vi "PicoScope5000aSettings.vi"(0 "error in":errorcluster, 1 "Channel A Settings":T2={"Enabled"=FALSE, "Coupling"=1, "Range"=6, "Analogue Offset"=0.0, "Bandwidth Limit"=0} {"Bandwidth Limit" items=["Full", "20MHz"]; "Range" items=["10 mV", "20 mV", "50 mV", "100 mV", "200 mV", "500 mV", "1 V", "2 V", "5 V", "10 V", "20 V"]; "Coupling" items=["AC", "DC"]}, 2 "Port 0 Settings":cluster{"Enabled":bool, "Logic Level":i16}={"Enabled"=FALSE, "Logic Level"=9830} {"Logic Level" items=["1.5V TTL"=9830, "2.5V CMOS"=16383]}, 3 "Channel B Settings":T2={"Enabled"=FALSE, "Coupling"=1, "Range"=6, "Analogue Offset"=0.0, "Bandwidth Limit"=0} {"Bandwidth Limit" items=["Full", "20MHz"]; "Range" items=["10 mV", "20 mV", "50 mV", "100 mV", "200 mV", "500 mV", "1 V", "2 V", "5 V", "10 V", "20 V"]; "Coupling" items=["AC", "DC"]}, 5 "handle in":i16, 9 "Device Info":T1, 11 "Trigger Settings":T3={"Trigger Enabled"=FALSE, "Trigger Source"=enum."Channel A", "Trigger Threshold (volts)"=0.0, "Trigger Direction"=2, "Trigger Delay (samples)"=0, "Auto Trigger Time (ms)"=1000} {"Trigger Direction" items=["Rising"=2, "Falling"=3]}, 12 "Channel C Settings":T2={"Enabled"=FALSE, "Coupling"=1, "Range"=6, "Analogue Offset"=0.0, "Bandwidth Limit"=0} {"Bandwidth Limit" items=["Full", "20MHz"]; "Range" items=["10 mV", "20 mV", "50 mV", "100 mV", "200 mV", "500 mV", "1 V", "2 V", "5 V", "10 V", "20 V"]; "Coupling" items=["AC", "DC"]}, 13 "Port 1 Settings":cluster{"Enabled":bool, "Logic Level":i16}={"Enabled"=FALSE, "Logic Level"=9830} {"Logic Level" items=["1.5V TTL"=9830, "2.5V CMOS"=16383]}, 14 "Channel D Settings":T2={"Enabled"=FALSE, "Coupling"=1, "Range"=6, "Analogue Offset"=0.0, "Bandwidth Limit"=0} {"Bandwidth Limit" items=["Full", "20MHz"]; "Range" items=["10 mV", "20 mV", "50 mV", "100 mV", "200 mV", "500 mV", "1 V", "2 V", "5 V", "10 V", "20 V"]; "Coupling" items=["AC", "DC"]}, 15 "Max ADC value":i16) -> (4 "error out":errorcluster, 6 "handle out":i16, 8 "enabled array":i16[](array[numeric]))   [LabVIEW 2020]
doc: "This VI is used to set up the oscilloscope. The inputs are clusters for setting channel and simple trigger settings. Advanced triggers can be set up using PicoScope3000aAdvancedTriggerSettings.vi"
uses:
  ps5000a.dll
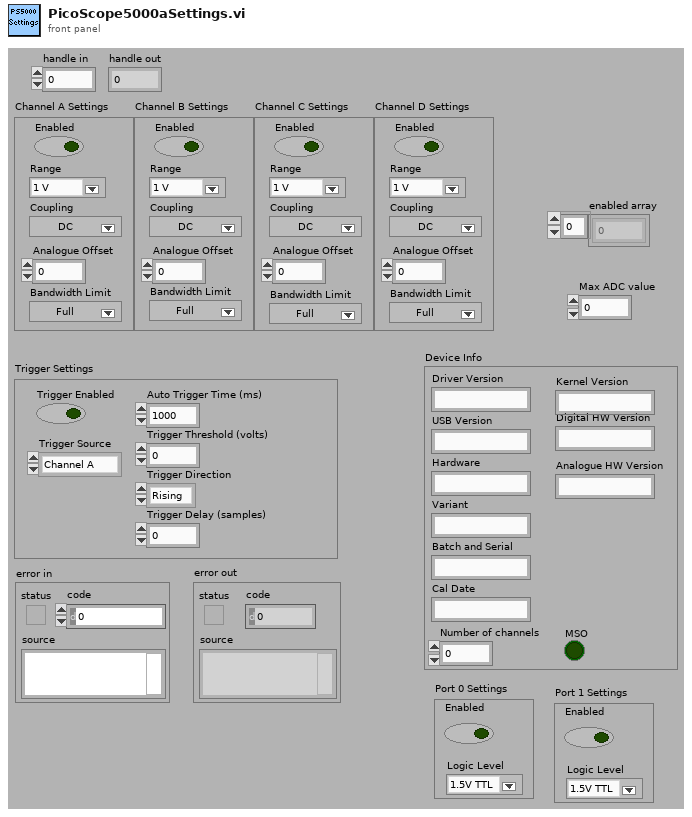
[diagram p1: front panel]
types:
  T1 = cluster{"Driver Version":string, "USB Version":string, "Hardware":string, "Variant":string, "Batch and Serial":string, "Cal Date":string, "Kernel Version":string, "Digital HW Version":string, "Analogue HW Version":string, "MSO":bool, "Number of channels":i16}
  T2 = cluster{"Enabled":bool, "Coupling":i16, "Range":u16, "Analogue Offset":sgl, "Bandwidth Limit":u32}
  T3 = cluster{"Trigger Enabled":bool, "Trigger Source":enum16{"Channel A", "Channel B", "Channel C", "Channel D", "Ext."}, "Trigger Threshold (volts)":dbl, "Trigger Direction":u16, "Trigger Delay (samples)":u32, "Auto Trigger Time (ms)":i16}
  T4 = enum16{"Channel A", "Channel B", "Channel C", "Channel D", "Ext."}
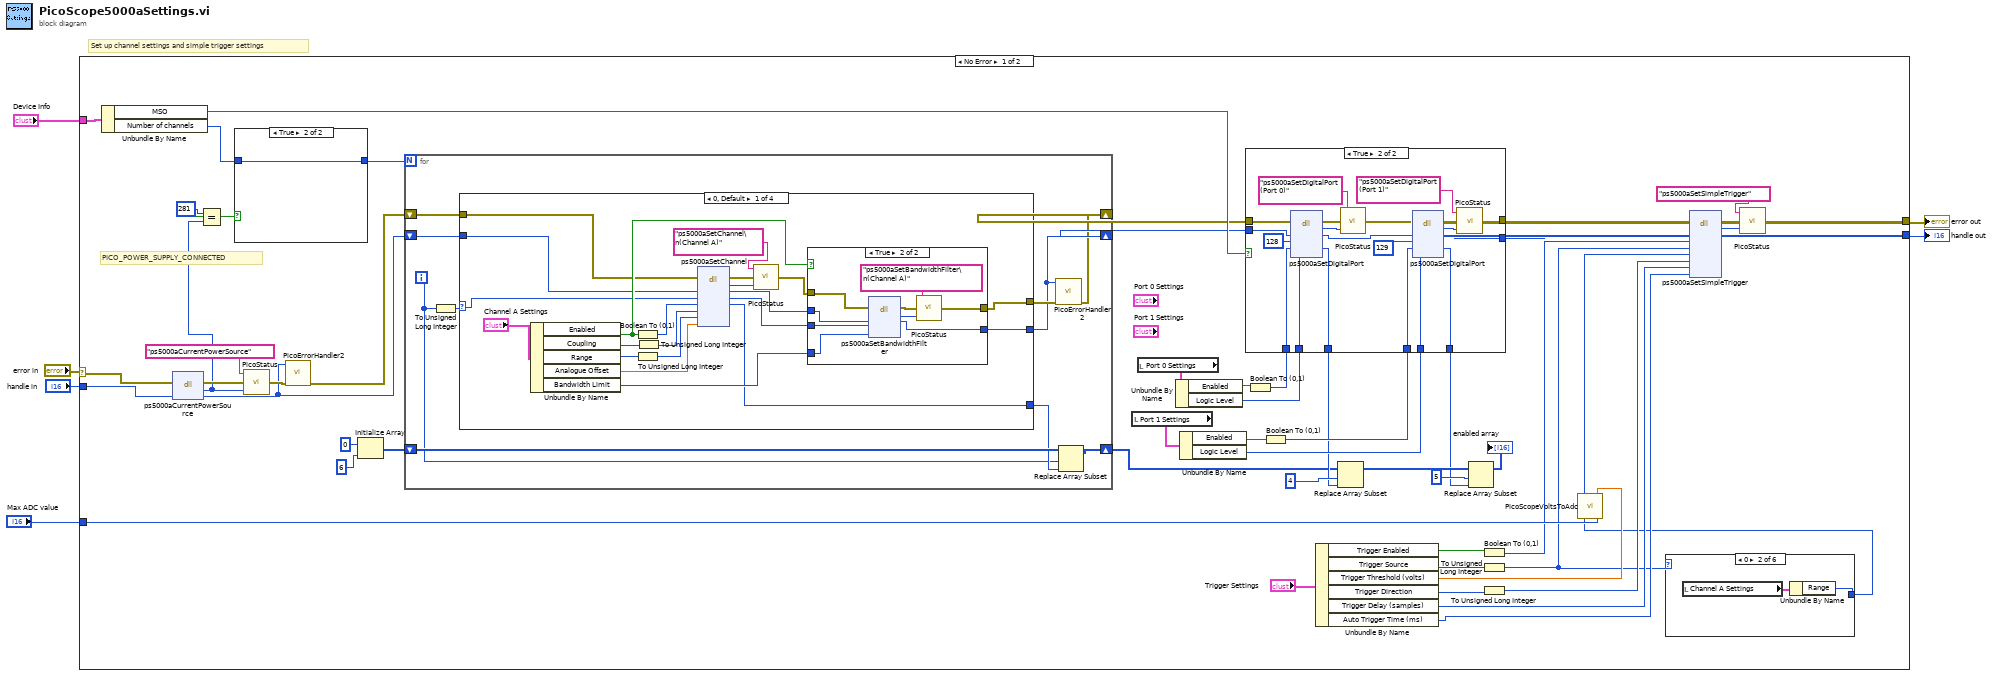
[diagram p0: block diagram]
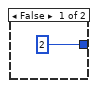
[diagram p2: hidden frame]
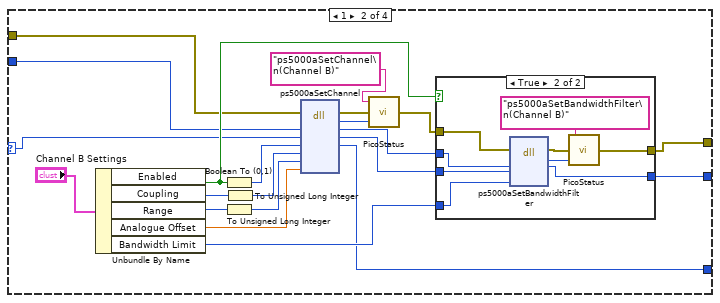
[diagram p4: hidden frame]
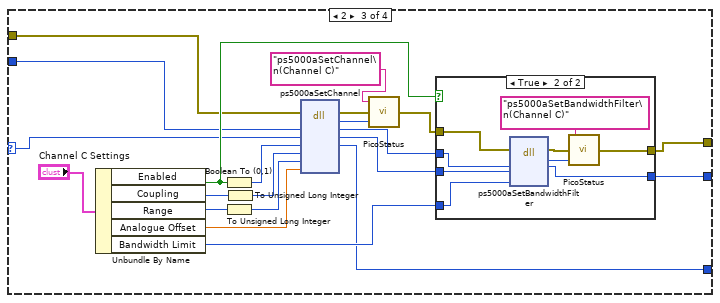
[diagram p6: hidden frame]
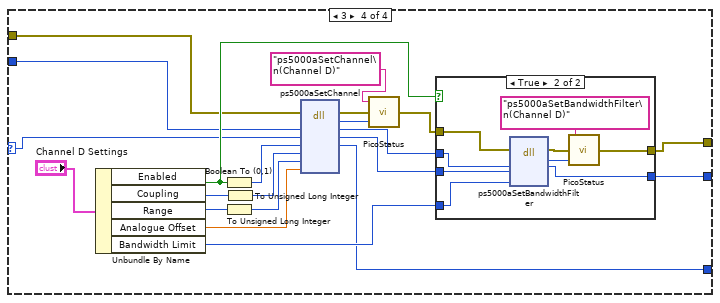
[diagram p8: hidden frame]
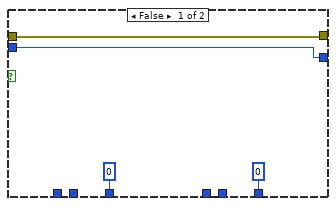
[diagram p10: hidden frame]
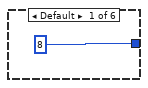
[diagram p11: hidden frame]
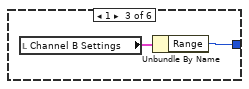
[diagram p12: hidden frame]
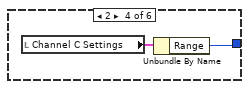
[diagram p13: hidden frame]
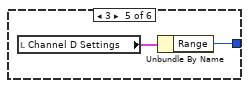
[diagram p14: hidden frame]
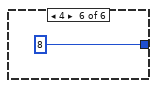
[diagram p15: hidden frame]
diagram:
  # "Set up channel settings and simple trigger settings"
  n1 = case shown="No Error" "error in" {
    selector: "error in" -> [w15 w236]
    tunnel: "handle in" -> [w14 w235]
    tunnel: [w51 w235] -> w4
    tunnel: [w40 w236] -> w3
    tunnel: "Device Info" -> [w46 _]
    tunnel: "Max ADC value" -> [w43 _]
    frame No Error {
      # "PICO_POWER_SUPPLY_CONNECTED"
      n2 = Unbundle By Name(w46) -> ("MSO"=w22:bool, "Number of channels"=w8:i16)
      n3 = dll-call lib="ps5000a.dll" fn="ps5000aCurrentPowerSource"(error in=w15, "handle"=w14) -> (error out=w49:errorcluster, "PICO_STATUS"=w47:u32, "handle"=w12:i16)  [unwired: 2 in, 1 out]
      n4 = Equal?(x=u32 281, y=w47) -> (x = y?=w10:bool)
      n5 = case shown="True" w10 {
        tunnel: [i16 2 ("Number of channels") w62] -> w9
        tunnel: w8 -> [_ w62]
        frame False {
        }
        frame True {
        }
      }
      n6 = call "PicoStatus.vi"("PICO STATUS"=w47, "error in"=w49, "source"="ps5000aCurrentPowerSource") -> ("error out"=w13:errorcluster)
      n7 = call "PicoErrorHandler2.vi"("error in (no error)"=w13, "handle In"=w12) -> ("error out"=w11:errorcluster)  [unwired: 9 in]
      n8 = Initialize Array(i16 0 ("element"), 6 ("dimension size")) -> (w19:i16[])
      n9 = for {
        N: w9 -> [_]
        shift-right: [w70] -> w18
        shift-left: w19 -> [w72]
        shift-right: [w67] -> w17
        shift-left: w11 -> [w69]
        shift-right: [w65] -> w16
        shift-left: w12 -> [w68]
        i -> [w63]
        n10 = To Unsigned Long Integer(number=w63) -> (unsigned 32bit integer=w64:u32)
        n11 = case shown="0, Default" w64 {
          selector: w64 -> [w73 w105 w137 w169]
          tunnel: [w78 w111 w143 w175] -> w71
          tunnel: w69 -> [w77 w109 w141 w173]
          tunnel: w68 -> [w76 w108 w140 w172]
          tunnel: [w75 w107 w139 w171] -> w66
          tunnel: [w74 w106 w138 w170] -> w65
          frame 0, Default {
            n12 = Unbundle By Name("Channel A Settings") -> ("Enabled"=w82:bool, "Coupling"=w92:i16, "Range"=w93:u16, "Analogue Offset"=w90:sgl, "Bandwidth Limit"=w83:u32)
            n13 = Boolean To (0,1)(Boolean=w82) -> (0, 1=w85:i16)
            n14 = To Unsigned Long Integer(number=w93) -> (unsigned 32bit integer=w89:u32)
            n15 = To Unsigned Long Integer(number=w92) -> (unsigned 32bit integer=w91:u32)
            n16 = dll-call lib="ps5000a.dll" fn="ps5000aSetChannel" ("ps3000.dll:_ps3000_open_unit@0")(error in=w77, "handle"=w76, "channel"=w73, "enabled"=w85, "dc"=w91, "range"=w89, "analogueOffset"=w90) -> (error out=w88:errorcluster, "PICO_STATUS"=w87:u32, "handle"=w80:i16, "channel"=w79:u32, "enabled"=w78:i16)  [unwired: 5 in, 1 out]
            n17 = call "PicoStatus.vi"("PICO STATUS"=w87, "error in"=w88, "source"="ps5000aSetChannel\n(Channel A)") -> ("error out"=w81:errorcluster)
            n18 = case shown="True" w82 {
              tunnel: w81 -> [w95 w101]
              tunnel: [w95 w100] -> w75
              tunnel: [w94 w99] -> w74
              tunnel: w79 -> [_ w98]
              tunnel: w80 -> [w94 w97]
              tunnel: w83 -> [_ w96]
              frame False {
              }
              frame True {
                n19 = dll-call lib="ps5000a.dll" fn="ps5000aSetBandwidthFilter" ("ps3000.dll:_ps3000_open_unit@0")(error in=w101, "handle"=w97, "channel"=w98, "Bandwidth Limit"=w96) -> (error out=w103:errorcluster, "PICO_STATUS"=w102:u32, "handle"=w99:i16)  [unwired: 4 in, 1 out]
                n20 = call "PicoStatus.vi"("PICO STATUS"=w102, "error in"=w103, "source"="ps5000aSetBandwidthFilter\n(Channel A)") -> ("error out"=w100:errorcluster)
              }
            }
          }
          frame 1 {
            n21 = Unbundle By Name("Channel B Settings") -> ("Enabled"=w115:bool, "Coupling"=w124:i16, "Range"=w125:u16, "Analogue Offset"=w122:sgl, "Bandwidth Limit"=w116:u32)
            n22 = Boolean To (0,1)(Boolean=w115) -> (0, 1=w118:i16)
            n23 = To Unsigned Long Integer(number=w125) -> (unsigned 32bit integer=w121:u32)
            n24 = To Unsigned Long Integer(number=w124) -> (unsigned 32bit integer=w123:u32)
            n25 = dll-call lib="ps5000a.dll" fn="ps5000aSetChannel" ("ps3000.dll:_ps3000_open_unit@0")(error in=w109, "handle"=w108, "channel"=w105, "enabled"=w118, "dc"=w123, "range"=w121, "analogueOffset"=w122) -> (error out=w120:errorcluster, "PICO_STATUS"=w119:u32, "handle"=w113:i16, "channel"=w112:u32, "enabled"=w111:i16)  [unwired: 5 in, 1 out]
            n26 = call "PicoStatus.vi"("PICO STATUS"=w119, "error in"=w120, "source"="ps5000aSetChannel\n(Channel B)") -> ("error out"=w114:errorcluster)
            n27 = case shown="True" w115 {
              tunnel: w114 -> [w127 w133]
              tunnel: [w127 w132] -> w107
              tunnel: [w126 w131] -> w106
              tunnel: w112 -> [_ w130]
              tunnel: w113 -> [w126 w129]
              tunnel: w116 -> [_ w128]
              frame False {
              }
              frame True {
                n28 = dll-call lib="ps5000a.dll" fn="ps5000aSetBandwidthFilter" ("ps3000.dll:_ps3000_open_unit@0")(error in=w133, "handle"=w129, "channel"=w130, "Bandwidth Limit"=w128) -> (error out=w135:errorcluster, "PICO_STATUS"=w134:u32, "handle"=w131:i16)  [unwired: 4 in, 1 out]
                n29 = call "PicoStatus.vi"("PICO STATUS"=w134, "error in"=w135, "source"="ps5000aSetBandwidthFilter\n(Channel B)") -> ("error out"=w132:errorcluster)
              }
            }
          }
          frame 2 {
            n30 = Unbundle By Name("Channel C Settings") -> ("Enabled"=w147:bool, "Coupling"=w156:i16, "Range"=w157:u16, "Analogue Offset"=w154:sgl, "Bandwidth Limit"=w148:u32)
            n31 = Boolean To (0,1)(Boolean=w147) -> (0, 1=w150:i16)
            n32 = To Unsigned Long Integer(number=w157) -> (unsigned 32bit integer=w153:u32)
            n33 = To Unsigned Long Integer(number=w156) -> (unsigned 32bit integer=w155:u32)
            n34 = dll-call lib="ps5000a.dll" fn="ps5000aSetChannel" ("ps3000.dll:_ps3000_open_unit@0")(error in=w141, "handle"=w140, "channel"=w137, "enabled"=w150, "dc"=w155, "range"=w153, "analogueOffset"=w154) -> (error out=w152:errorcluster, "PICO_STATUS"=w151:u32, "handle"=w145:i16, "channel"=w144:u32, "enabled"=w143:i16)  [unwired: 5 in, 1 out]
            n35 = call "PicoStatus.vi"("PICO STATUS"=w151, "error in"=w152, "source"="ps5000aSetChannel\n(Channel C)") -> ("error out"=w146:errorcluster)
            n36 = case shown="True" w147 {
              tunnel: w146 -> [w159 w165]
              tunnel: [w159 w164] -> w139
              tunnel: [w158 w163] -> w138
              tunnel: w144 -> [_ w162]
              tunnel: w145 -> [w158 w161]
              tunnel: w148 -> [_ w160]
              frame False {
              }
              frame True {
                n37 = dll-call lib="ps5000a.dll" fn="ps5000aSetBandwidthFilter" ("ps3000.dll:_ps3000_open_unit@0")(error in=w165, "handle"=w161, "channel"=w162, "Bandwidth Limit"=w160) -> (error out=w167:errorcluster, "PICO_STATUS"=w166:u32, "handle"=w163:i16)  [unwired: 4 in, 1 out]
                n38 = call "PicoStatus.vi"("PICO STATUS"=w166, "error in"=w167, "source"="ps5000aSetBandwidthFilter\n(Channel C)") -> ("error out"=w164:errorcluster)
              }
            }
          }
          frame 3 {
            n39 = Unbundle By Name("Channel D Settings") -> ("Enabled"=w179:bool, "Coupling"=w188:i16, "Range"=w189:u16, "Analogue Offset"=w186:sgl, "Bandwidth Limit"=w180:u32)
            n40 = Boolean To (0,1)(Boolean=w179) -> (0, 1=w182:i16)
            n41 = To Unsigned Long Integer(number=w189) -> (unsigned 32bit integer=w185:u32)
            n42 = To Unsigned Long Integer(number=w188) -> (unsigned 32bit integer=w187:u32)
            n43 = dll-call lib="ps5000a.dll" fn="ps5000aSetChannel" ("ps3000.dll:_ps3000_open_unit@0")(error in=w173, "handle"=w172, "channel"=w169, "enabled"=w182, "dc"=w187, "range"=w185, "analogueOffset"=w186) -> (error out=w184:errorcluster, "PICO_STATUS"=w183:u32, "handle"=w177:i16, "channel"=w176:u32, "enabled"=w175:i16)  [unwired: 5 in, 1 out]
            n44 = call "PicoStatus.vi"("PICO STATUS"=w183, "error in"=w184, "source"="ps5000aSetChannel\n(Channel D)") -> ("error out"=w178:errorcluster)
            n45 = case shown="True" w179 {
              tunnel: w178 -> [w191 w197]
              tunnel: [w191 w196] -> w171
              tunnel: [w190 w195] -> w170
              tunnel: w176 -> [_ w194]
              tunnel: w177 -> [w190 w193]
              tunnel: w180 -> [_ w192]
              frame False {
              }
              frame True {
                n46 = dll-call lib="ps5000a.dll" fn="ps5000aSetBandwidthFilter" ("ps3000.dll:_ps3000_open_unit@0")(error in=w197, "handle"=w193, "channel"=w194, "Bandwidth Limit"=w192) -> (error out=w199:errorcluster, "PICO_STATUS"=w198:u32, "handle"=w195:i16)  [unwired: 4 in, 1 out]
                n47 = call "PicoStatus.vi"("PICO STATUS"=w198, "error in"=w199, "source"="ps5000aSetBandwidthFilter\n(Channel D)") -> ("error out"=w196:errorcluster)
              }
            }
          }
        }
        n48 = call "PicoErrorHandler2.vi"("error in (no error)"=w66, "handle In"=w65) -> ("error out"=w67:errorcluster)  [unwired: 9 in]
        n49 = Replace Array Subset(array=w72, new element=w71, index=w63) -> (w70:i16[])
      }
      n50 = local read "Port 1 Settings"() -> (w38:cluster{"Enabled":bool, "Logic Level":i16})
      n51 = local read "Port 0 Settings"() -> (w39:cluster{"Enabled":bool, "Logic Level":i16})
      n52 = Unbundle By Name(w39) -> ("Enabled"=w37:bool, "Logic Level"=w35:i16)
      n53 = Unbundle By Name(w38) -> ("Enabled"=w34:bool, "Logic Level"=w32:i16)
      n54 = Boolean To (0,1)(Boolean=w37) -> (0, 1=w36:i16)
      n55 = Boolean To (0,1)(Boolean=w34) -> (0, 1=w33:i16)
      n56 = case shown="True" w22 {
        tunnel: [w204 w216] -> w31
        tunnel: w36 -> [_ w213]
        tunnel: w35 -> [_ w212]
        tunnel: w33 -> [_ w211]
        tunnel: w32 -> [_ w210]
        tunnel: w17 -> [w204 w209]
        tunnel: w16 -> [w203 w208]
        tunnel: [w203 w207] -> w30
        tunnel: [i16 0 ("enabled") w206] -> w25
        tunnel: [i16 0 ("enabled") w205] -> w24
        frame False {
        }
        frame True {
          n57 = dll-call lib="PS5000a.dll" fn="ps5000aSetDigitalPort"(error in=w209, "handle"=w208, "port"=u32 128, "enabled"=w213, "logicLevel"=w212) -> (error out=w224:errorcluster, "PICO_STATUS"=w221:u32, "handle"=w217:i16, "enabled"=w206:i16)  [unwired: 4 in, 1 out]
          n58 = call "PicoStatus.vi"("PICO STATUS"=w221, "error in"=w224, "source"="ps5000aSetDigitalPort (Port 0)") -> ("error out"=w218:errorcluster)
          n59 = dll-call lib="PS5000a.dll" fn="ps5000aSetDigitalPort"(error in=w218, "handle"=w217, "port"=u32 129, "enabled"=w211, "logicLevel"=w210) -> (error out=w220:errorcluster, "PICO_STATUS"=w219:u32, "handle"=w207:i16, "enabled"=w205:i16)  [unwired: 4 in, 1 out]
          n60 = call "PicoStatus.vi"("PICO STATUS"=w219, "error in"=w220, "source"="ps5000aSetDigitalPort (Port 1)") -> ("error out"=w216:errorcluster)
        }
      }
      n61 = Unbundle By Name("Trigger Settings") -> ("Trigger Enabled"=w55:bool, "Trigger Source"=w56:T4, "Trigger Threshold (volts)"=w44:dbl, "Trigger Direction"=w58:u16, "Trigger Delay (samples)"=w57:u32, "Auto Trigger Time (ms)"=w42:i16)
      n62 = Replace Array Subset(array=w18, new element=w25, index=4) -> (w26:i16[])
      n63 = Replace Array Subset(array=w26, new element=w24, index=5) -> (→"enabled array":i16[])
      n64 = Boolean To (0,1)(Boolean=w55) -> (0, 1=w29:i16)
      n65 = To Unsigned Long Integer(number=w56) -> (unsigned 32bit integer=w41:u32)
      n66 = To Unsigned Long Integer(number=w58) -> (unsigned 32bit integer=w60:u32)
      n67 = case shown="0" w41 {
        tunnel: [u16 8 ("Range") w226 w228 w230 w232 u16 8 ("Range")] -> w7
        frame Default {
        }
        frame 0 {
          n68 = local read "Channel A Settings"() -> (w227:T2)
          n69 = Unbundle By Name(w227) -> ("Range"=w226:u16)
        }
        frame 1 {
          n70 = local read "Channel B Settings"() -> (w229:T2)
          n71 = Unbundle By Name(w229) -> ("Range"=w228:u16)
        }
        frame 2 {
          n72 = local read "Channel C Settings"() -> (w231:T2)
          n73 = Unbundle By Name(w231) -> ("Range"=w230:u16)
        }
        frame 3 {
          n74 = local read "Channel D Settings"() -> (w233:T2)
          n75 = Unbundle By Name(w233) -> ("Range"=w232:u16)
        }
        frame 4 {
        }
      }
      n76 = call "PicoScopeVoltsToAdc.vi"("Max_adc"=w43, "Volts"=w44, "Range Index"=w7) -> ("ADC count"=w45:i16)
      n77 = dll-call lib="ps5000a.dll" fn="ps5000aSetSimpleTrigger" ("ps3000.dll:_ps3000_open_unit@0")(error in=w31, "handle"=w30, "enable"=w29, "source"=w41, "threshold"=w45, "direction"=w60, "delay"=w57, "autoTrigger_ms"=w42) -> (error out=w53:errorcluster, "PICO_STATUS"=w54:u32, "handle"=w51:i16)  [unwired: 8 in, 1 out]
      n78 = call "PicoStatus.vi"("PICO STATUS"=w54, "error in"=w53, "source"="ps5000aSetSimpleTrigger") -> ("error out"=w40:errorcluster)
    }
    frame Error {
    }
  }
  "handle out" <- w4
  "error out" <- w3
